vi "Experiment header-Get file name.vi"(8 "error in (no error)":errorcluster, 11 "Experiment data folder path":path) -> (0 "error out":errorcluster, 3 "Header File Path":path)   [LabVIEW 2017]
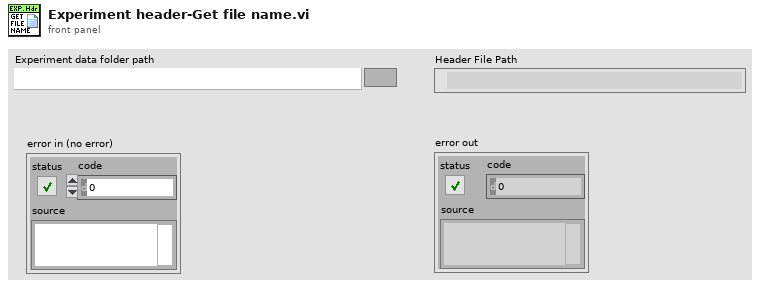
[diagram p1: front panel]
types:
  T1 = typedef "Fixed strings.ctl" = cluster{"ROI file name":string, "Normalised ROI file name":string, "Zplane Pockels values file name":string, "Functional data folder name":string, "Experiment Header file name":string, "Z-stack images folder name":string, "Groups setup rel. path":string, "Groups text file rel. path":string, "TDMS files folder name (F.img)":string, "TDMS files folder name (V.acq)":string, "TDMS files folder name (Pl.acq)":string, "Cycle rel times sequence file":string, "Dynamically called VIs folder name":string, "Time Series folder base name":string}
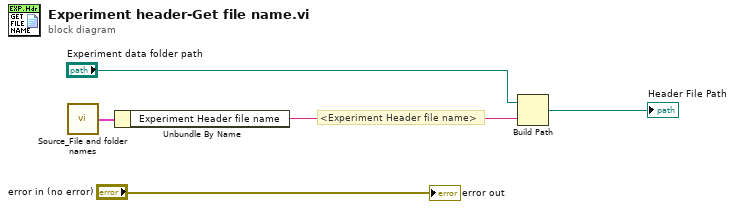
[diagram p0: block diagram]
diagram:
  # "<Experiment Header file name>"
  n1 = call "Source_File and folder names.vi"() -> ("Fixed strings"=w5:T1)  [unwired: 1 in]
  n2 = Unbundle By Name(w5) -> ("Experiment Header file name"=w4:string)
  n3 = Build Path(base path="Experiment data folder path", name or relative path=w4) -> (appended path=→"Header File Path":path)
  "error out" <- "error in (no error)"
